vi "Config File View SubVI.vi"(10 "Config file view":bool, 11 "Path in":refnum<vi>) -> (2 "concatenated string":string, 3 "data":T1(array[cluster]))   [LabVIEW 2019]
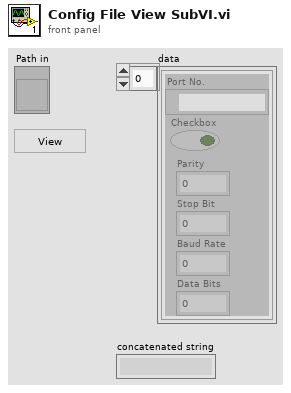
[diagram p1: front panel]
types:
  T1 = cluster{"Port No.":refnum<visa-resource-name>, "Checkbox":bool, "Parity":u16, "Stop Bit":u16, "Baud Rate":dbl, "Data Bits":dbl}[]
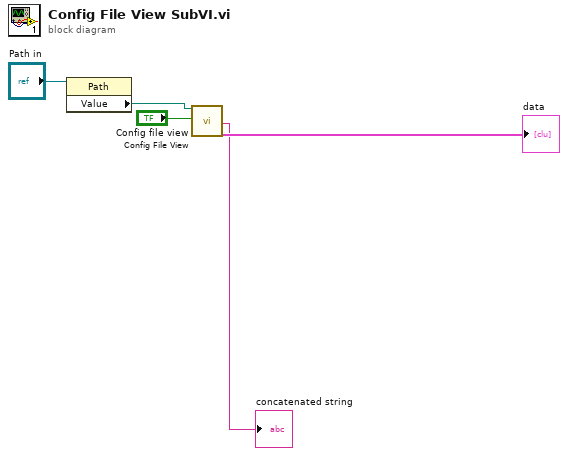
[diagram p0: block diagram]
diagram:
  n1 = property class="Path"(reference="Path in") -> ("Value"=w3:path)  [unwired: 1 in, 2 out]
  n2 = call "Config File View.vi"("Path"=w3, "File View"="Config file view") -> ("concatenated string"=→"concatenated string":string, "data"=→"data":T1)  [unwired: 16 in]
